vi "Can_Remove_Build_Output_On_Error.vi"(8 "error in (no error)":errorcluster, 11 "Build in":refnum<class "AB_PackedLibrary.lvclass">) -> (0 "error out":errorcluster, 2 "Remove build output":bool, 3 "Build out":refnum<class "AB_PackedLibrary.lvclass">)   [LabVIEW 2020, in "AB_PackedLibrary.lvclass"]
uses:
  <vilib>/AppBuilder/AB_Classes/PackedLib/AB_PackedLibrary.lvclass
  <vilib>/AppBuilder/AB_Classes/PackedLib/AB_PackedLibrary.lvclass/AB_PackedLibrary.ctl
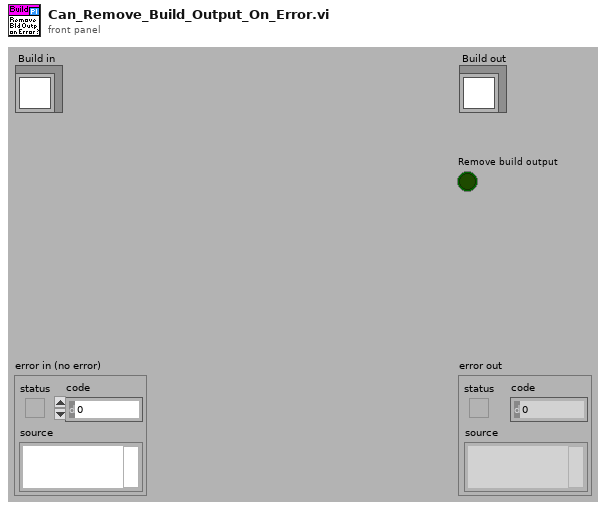
[diagram p1: front panel]
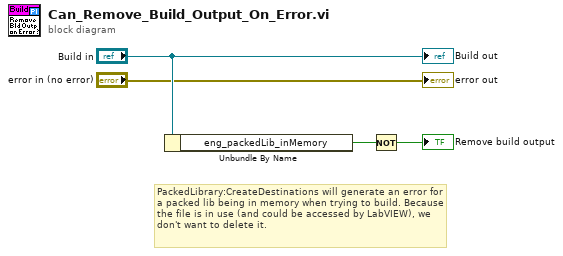
[diagram p0: block diagram]
diagram:
  # "PackedLibrary:CreateDestinations will generate an error for a packed lib being in memory when trying to build. Because the file is in use (and could be accessed by LabVIEW), we don't want to delete it."
  n1 = Unbundle By Name("Build in") -> ("eng_packedLib_inMemory"=w4:bool)
  n2 = Not(x=w4) -> (.not. x?=→"Remove build output":bool)
  "error out" <- "error in (no error)"
  "Build out" <- "Build in"
